vi "initial_config.vi"(8 "error in (no error)":errorcluster, 11 "config_file_name":string="reg_service_config.ini") -> (0 "error out":errorcluster, 3 "Data":T1)   [LabVIEW 2015]
doc: "This vi does the following tasks: \n1.- Create the Test Log folder and subfolders, \n2.- Get the timeout values from config file, \n3.- Get the endpoint address from config file,\n4.- Get the file extension to search (i.e *json) from config file.,\n5.- Get holding time from config file."
uses:
  typedef/init_config_data.ctl
  <vilib>/Utility/error.llb/Error Cluster From Error Code.vi
  <vilib>/ErrorRing/Error Ring.xnode
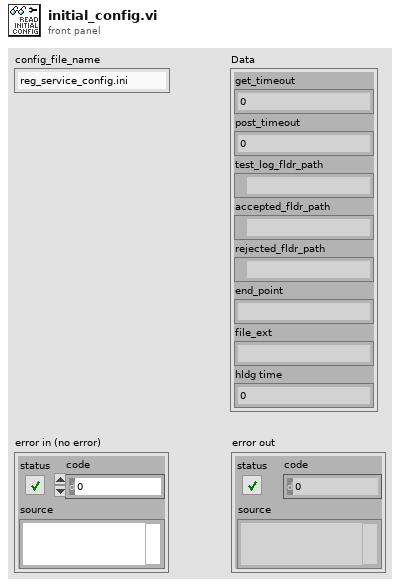
[diagram p1: front panel]
types:
  T1 = typedef "init_config_data.ctl" = cluster{"end_point":string, "file_ext":string, "hldg time":dbl, "test_log_fldr_path":path, "accepted_fldr_path":path, "rejected_fldr_path":path, "post_timeout":i32, "get_timeout":i32}
  T2 = cluster{"test_log_base_path":string, "accepted_folder_name":string, "rejected_folder_name":string}
  T3 = typedef "created_folders_path.ctl" = cluster{"test_log_fldr_path":path, "accepted_fldr_path":path, "rejected_fldr_path":path}
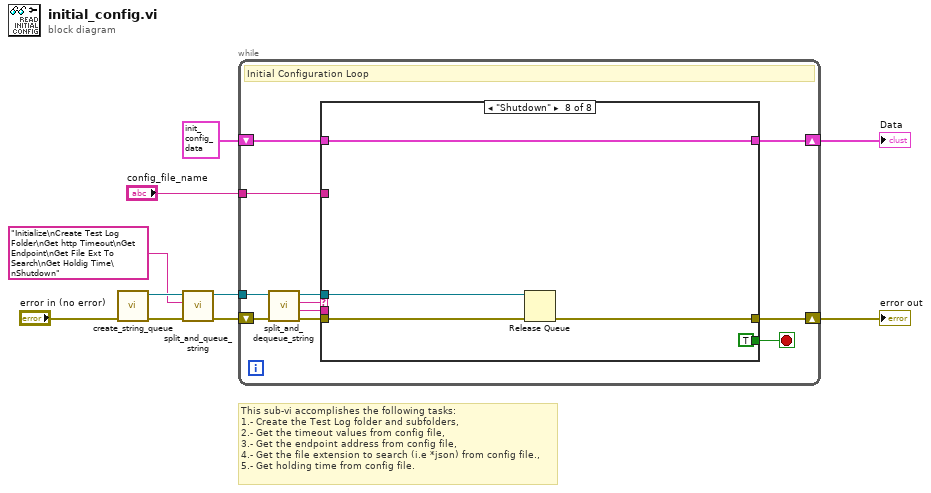
[diagram p0: block diagram]
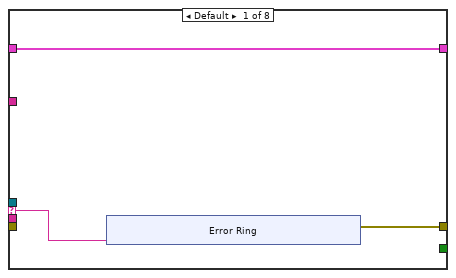
[diagram p2: hidden frame]
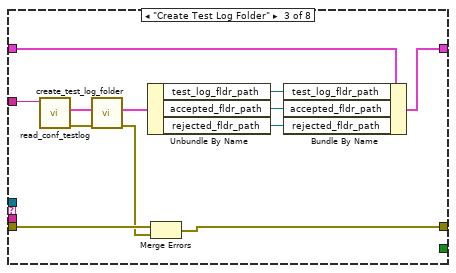
[diagram p4: hidden frame]
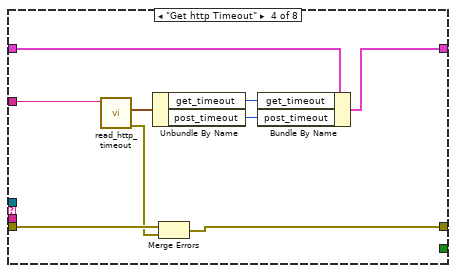
[diagram p5: hidden frame]
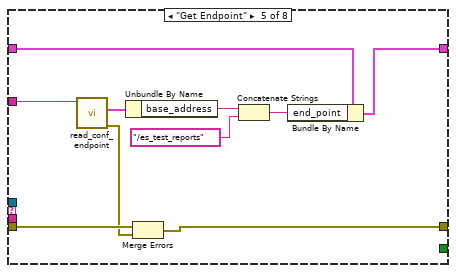
[diagram p6: hidden frame]
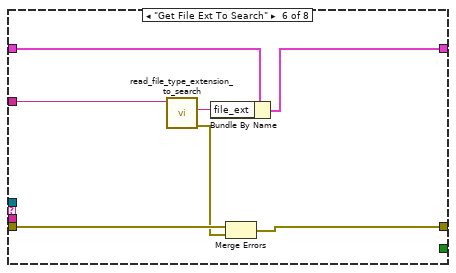
[diagram p7: hidden frame]
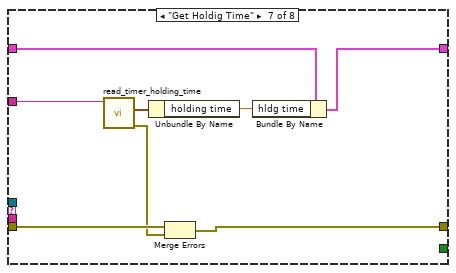
[diagram p8: hidden frame]
diagram:
  # "This sub-vi accomplishes the following tasks: \n1.- Create the Test Log folder and subfolders, \n2.- Get the timeout values from config file, \n3.- Get the endpoint address from config file,\n4.- Get the file extension to search (i.e *json) from config file.,\n5.- Get holding time from config file."
  n1 = call "create_string_queue.vi"("error in (no error)"="error in (no error)") -> ("error out"=w9:errorcluster, "Queue out"=w10:refnum<queue>)  [unwired: 9 in]
  n2 = call "split_and_queue_string.vi"("error in (no error)"=w9, "list state:argument"="Initialize\nCreate Test Log Folder\nGet http Timeout\nGet Endpoint\nGet File Ext To Search\nGet Holdig Time\nShutdown", "Queue in"=w10) -> ("error out"=w8:errorcluster, "Queue out"=w7:refnum<queue>)  [unwired: 7 in]
  n3 = while {
    shift-right: [w19] -> w5
    shift-left: w8 -> [w21]
    tunnel: w7 -> [w17]
    shift-right: [w13] -> w3
    shift-left: T1 {"end_point"="", "file_ext"="", "hldg time"=0.0, "test_log_fldr_path"=path "", "accepted_fldr_path"=path "", "rejected_fldr_path"=path "", "post_timeout"=0, "get_timeout"=0} ("Data") -> [w14]
    tunnel: "config_file_name" -> [w12]
    stop <- w18 stop-if-true
    # "Initial Configuration Loop"
    n4 = call "split_and_dequeue_string.vi"("error in (no error)"=w21, "Queue in"=w17) -> ("error out"=w20:errorcluster, "argument"=w15:string, "state"=w16:string, "Queue out"=w11:refnum<queue>)  [unwired: 6 in]
    n5 = case shown="\"Shutdown\"" w16 {
      selector: w16 -> [w23 _ _ _ _ _ _ _]
      tunnel: w20 -> [_ w33 w45 w54 w64 w71 w79 w83]
      tunnel: [w22 w33 w40 w50 w56 w68 w74 w81] -> w19
      tunnel: [_ _ _ _ _ _ _ TRUE] -> w18
      tunnel: w11 -> [_ _ _ _ _ _ _ w82]
      tunnel: w15 -> [_ _ _ _ _ _ _ _]
      tunnel: w12 -> [_ _ w43 w53 w59 w69 w76 _]
      tunnel: w14 -> [w24 w32 w42 w52 w58 w66 w75 w80]
      tunnel: [w24 w32 w41 w51 w57 w65 w72 w80] -> w13
      frame Default {
        n6 = xnode "Error Ring"("parameter 0"=w23) -> ("error out"=w22:errorcluster)
      }
      frame "Initialize" {
      }
      frame "Create Test Log Folder" {
        n7 = call "read_conf_testlog.vi"("config_file_name"=w43) -> ("error out"=w44:errorcluster, "values"=w35:T2)  [unwired: 8 in, 1 out]
        n8 = call "create_test_log_folder.vi"("error in (no error)"=w44, "names in"=w35) -> ("error out"=w39:errorcluster, "fldr paths"=w34:T3)  [unwired: 8 in]
        n9 = Unbundle By Name(w34) -> ("test_log_fldr_path"=w38:path, "accepted_fldr_path"=w37:path, "rejected_fldr_path"=w36:path)
        n10 = Merge Errors(w45, w39) -> (w40:errorcluster)
        n11 = Bundle By Name(cluster=w42, "test_log_fldr_path"=w38, "accepted_fldr_path"=w37, "rejected_fldr_path"=w36) -> (w41:T1)
      }
      frame "Get http Timeout" {
        n12 = call "read_http_timeout.vi"("config_file_name"=w53) -> ("error out"=w49:errorcluster, "values"=w48:cluster{"get_timeout":i32, "post_timeout":i32})  [unwired: 8 in, 1 out]
        n13 = Unbundle By Name(w48) -> ("get_timeout"=w47:i32, "post_timeout"=w46:i32)
        n14 = Merge Errors(w54, w49) -> (w50:errorcluster)
        n15 = Bundle By Name(cluster=w52, "get_timeout"=w47, "post_timeout"=w46) -> (w51:T1)
      }
      frame "Get Endpoint" {
        n16 = call "read_conf_endpoint.vi"("config_file_name"=w59) -> ("error out"=w55:errorcluster, "values"=w60:cluster{"base_address":string})  [unwired: 8 in, 1 out]
        n17 = Unbundle By Name(w60) -> ("base_address"=w61:string)
        n18 = Merge Errors(w64, w55) -> (w56:errorcluster)
        n19 = Concatenate Strings(w61, "/es_test_reports" ("string")) -> (w63:string)
        n20 = Bundle By Name(cluster=w58, "end_point"=w63) -> (w57:T1)
      }
      frame "Get File Ext To Search" {
        n21 = call "read_file_type_extension_to_search.vi"("config_file_name"=w69) -> ("error out"=w67:errorcluster, "extension_to_search"=w70:string)  [unwired: 8 in, 1 out]
        n22 = Bundle By Name(cluster=w66, "file_ext"=w70) -> (w65:T1)
        n23 = Merge Errors(w71, w67) -> (w68:errorcluster)
      }
      frame "Get Holdig Time" {
        n24 = call "read_timer_holding_time.vi"("config_file_name"=w76) -> ("error out"=w73:errorcluster, "values"=w77:cluster{"holding time":dbl})  [unwired: 8 in, 1 out]
        n25 = Unbundle By Name(w77) -> ("holding time"=w78:dbl)
        n26 = Merge Errors(w79, w73) -> (w74:errorcluster)
        n27 = Bundle By Name(cluster=w75, "hldg time"=w78) -> (w72:T1)
      }
      frame "Shutdown" {
        n28 = Release Queue(queue=w82, error in (no error)=w83) -> (error out=w81:errorcluster)  [unwired: 1 in, 2 out]
      }
    }
  }
  "error out" <- w5
  "Data" <- w3
